vi "SmartMotor_single motor update motion params and go.vi"(0 "VISA In":refnum<visa-resource-name>, 1 "Update? (T)":T2={"PosType"=TRUE, "Pos"=TRUE, "Vel"=TRUE, "Accel"=TRUE}, 2 "Cnts ScaleFactors":T5, 5 "motion params":T3={"PosType(Rel)"=enum."Relative", "Pos"=0.0, "Vel"=0.0, "Accel"=0.0}, 7 "MotorSpecifier(None)":T1, 9 "SendGo? (T)":bool=TRUE, 11 "error in":errorcluster, 12 "InterParamWait (5ms)":u32=5, 13 "ReadWait":u32=50, 14 "Semaphore Timeout (5000)":i32=5000) -> (4 "VISA out":refnum<visa-resource-name>, 6 "Cmd Str out":string, 15 "error out":errorcluster)   [LabVIEW 2017]
doc: "Developed by: Kevin Thompson\nThompson Engineering\nkevin@thompsonengineering.net\n(510) 673-3614"
uses:
  TD Cnts ScaleFactors - [EU to Cnts].ctl
  TD MotionParams--cluster.ctl
  TD PositionType_enum.ctl
  TD SelectMotionParamsUpdate--cluster.ctl
  TD SerialBusMotorSpecifier_enum.ctl
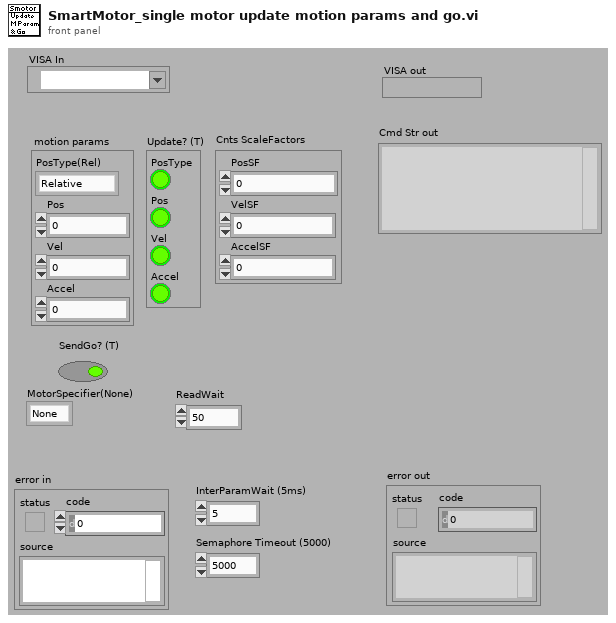
[diagram p1: front panel]
types:
  T1 = typedef "TD SerialBusMotorSpecifier_enum.ctl" = enum16{"None", "Global", "M1", "M2", "M3"}
  T2 = typedef "TD SelectMotionParamsUpdate--cluster.ctl" = cluster{"PosType":bool, "Pos":bool, "Vel":bool, "Accel":bool}
  T3 = typedef "TD MotionParams--cluster.ctl" = cluster{"PosType(Rel)":T4, "Pos":dbl, "Vel":dbl, "Accel":dbl}
  T4 = typedef "TD PositionType_enum.ctl" = enum16{"Absolute", "Relative"}
  T5 = typedef "TD Cnts ScaleFactors - [EU to Cnts].ctl" = cluster{"PosSF":dbl, "VelSF":dbl, "AccelSF":dbl}
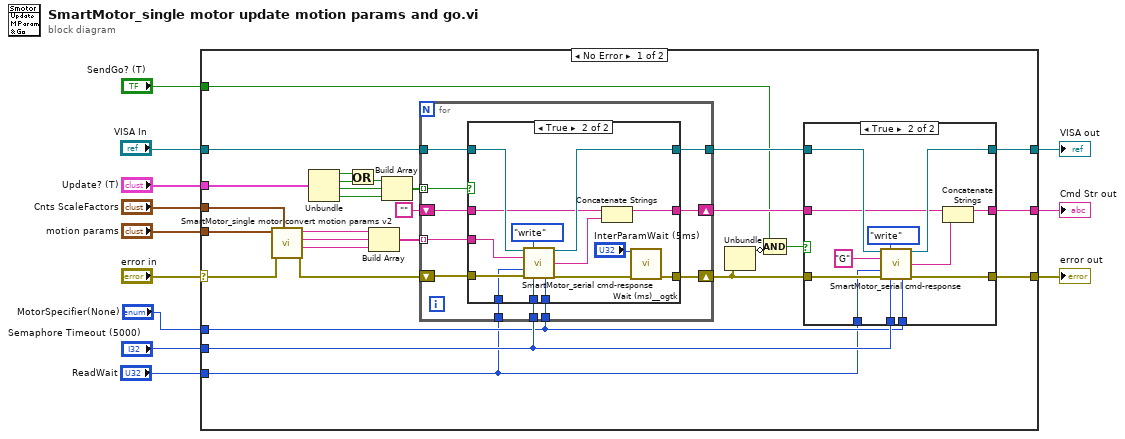
[diagram p0: block diagram]
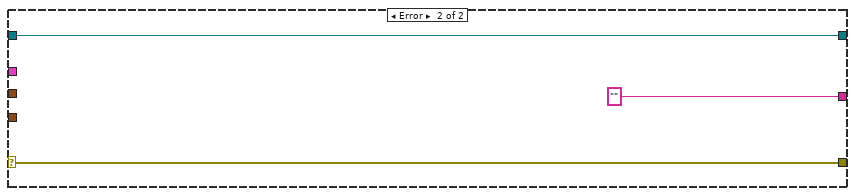
[diagram p4: hidden frame]
diagram:
  n1 = case shown="No Error" "error in" {
    selector: "error in" -> [w16 w86]
    tunnel: [w40 w86] -> w12
    tunnel: [w28 w87] -> w11
    tunnel: "VISA In" -> [w27 w87]
    tunnel: [w24 ""] -> w8
    tunnel: "motion params" -> [w18 _]
    tunnel: "Cnts ScaleFactors" -> [w21 _]
    tunnel: "Semaphore Timeout (5000)" -> [w20 _]
    tunnel: "SendGo? (T)" -> [w19 _]
    tunnel: "Update? (T)" -> [w17 _]
    tunnel: "MotorSpecifier(None)" -> [w14 _]
    tunnel: "ReadWait" -> [w13 _]
    frame No Error {
      n2 = call "SmartMotor_single motor convert motion params v2.vi"("Cnts ScaleFactors"=w21, "error in (no error)"=w16, "motion params"=w18) -> ("error out"=w15:errorcluster, "accelCmd"=w34:string, "velCmd"=w35:string, "posCmd"=w36:string)  [unwired: 5 in]
      n3 = Unbundle(w17) -> ("PosType"=w33:bool, "Pos"=w32:bool, "Vel"=w22:bool, "Accel"=w23:bool)
      n4 = Or(x=w33, y=w32) -> (x .or. y?=w31:bool)
      n5 = Build Array(w36, w35, w34) -> (w41:string[])
      n6 = Build Array(w31, w22, w23) -> (w30:bool[])
      n7 = for {
        tunnel: w41 -> [w67] mode=indexing
        tunnel: w30 -> [w59] mode=indexing
        shift-right: [w66] -> w39
        shift-left: w15 -> [w65]
        tunnel: w27 -> [w64]
        tunnel: [w63] -> w29
        tunnel: w20 -> [w62]
        shift-right: [w60] -> w25
        shift-left: "" -> [w61]
        tunnel: w14 -> [w58]
        tunnel: w13 -> [w57]
        n8 = case shown="True" w59 {
          tunnel: w67 -> [_ w84]
          tunnel: [w70 w81] -> w66
          tunnel: w65 -> [w70 w79]
          tunnel: w64 -> [w69 w78]
          tunnel: [w69 w77] -> w63
          tunnel: w62 -> [_ w76]
          tunnel: w61 -> [w68 w75]
          tunnel: [w68 w73] -> w60
          tunnel: w58 -> [_ w72]
          tunnel: w57 -> [_ w71]
          frame False {
          }
          frame True {
            n9 = call "SmartMotor_serial cmd-response.vi"("VISA In"=w78, "mode"=enum16{"wr & rd", "write", "read"}."write", "cmd"=w84, "ReadWait"=w71, "error in"=w79, "Sem Timeout (5000)"=w76, "MotorSpecifier(None)"=w72) -> ("VISA out"=w77:refnum<visa-resource-name>, "cmd str out"=w74:string, "error out"=w82:errorcluster)  [unwired: 4 in, 2 out]
            n10 = Concatenate Strings(w75, w74) -> (w73:string)
            n11 = call <userlib>:"Wait (ms)__ogtk.vi"("error in (no error)"=w82, "milliseconds to wait"="InterParamWait (5ms)") -> ("error out"=w81:errorcluster)  [unwired: 8 in, 1 out]
          }
        }
      }
      n12 = Unbundle(w39) -> ("status"=w38:bool)  [unwired: 2 out]
      n13 = Compound Arithmetic op=AND(w19, invert w38) -> (w37:bool)
      n14 = case shown="True" w37 {
        tunnel: w39 -> [w44 w55]
        tunnel: [w44 w54] -> w40
        tunnel: w29 -> [w43 w52]
        tunnel: [w43 w51] -> w28
        tunnel: w20 -> [_ w50]
        tunnel: w25 -> [w42 w49]
        tunnel: [w42 w47] -> w24
        tunnel: w14 -> [_ w46]
        tunnel: w13 -> [_ w45]
        frame False {
        }
        frame True {
          n15 = call "SmartMotor_serial cmd-response.vi"("VISA In"=w52, "mode"=enum16{"wr & rd", "write", "read"}."write", "cmd"="G" ("String to Write"), "ReadWait"=w45, "error in"=w55, "Sem Timeout (5000)"=w50, "MotorSpecifier(None)"=w46) -> ("VISA out"=w51:refnum<visa-resource-name>, "cmd str out"=w48:string, "error out"=w54:errorcluster)  [unwired: 4 in, 2 out]
          n16 = Concatenate Strings(w49, w48) -> (w47:string)
        }
      }
    }
    frame Error {
    }
  }
  "error out" <- w12
  "VISA out" <- w11
  "Cmd Str out" <- w8
